vi "tm_errorreport.vi"(1 "Source":path, 2 "Error":i32) -> (0 "error out":errorcluster {"code" format="%.0x"})   [LabVIEW 2015]
uses:
  tmcamcon.dll
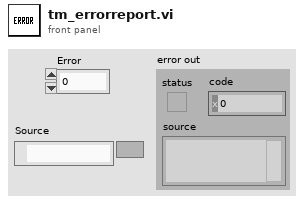
[diagram p1: front panel]
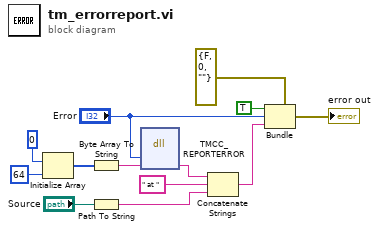
[diagram p0: block diagram]
diagram:
  n1 = Initialize Array(u8 0, 64) -> (w6:u8[])
  n2 = Byte Array To String(unsigned byte array=w6) -> (string=w5:string)
  n3 = Path To String(path="Source") -> (string=w4:string)
  n4 = dll-call lib="tmcamcon.dll" fn="TMCC_REPORTERROR"("error"="Error", "Erval"=w5) -> ("Erval"=w9:string)  [unwired: 5 in, 2 out]
  n5 = Concatenate Strings(w9, " at ", w4) -> (w2:string)
  n6 = Bundle(cluster=cluster{"status":bool, "Erval":i32, string} {"status"=FALSE, "Erval"=0, ""}, "status"=TRUE, "Erval"="Error", w2) -> (→"error out":cluster{"status":bool, "Erval":i32, string})
